vi "Read Host Stream.vi"(5 "Pause":bool, 7 "Init?":bool, 8 "error in (no error)":errorcluster, 10 "Sort By ID":bool, 11 "Refs in":T2) -> (0 "error out":errorcluster, 2 "Stream":T1, 3 "Refs out":T2)   [LabVIEW 2019, in "CAN Streaming Support Workspace Shared.lvlib"]
uses:
  CAN Streaming Support Workspace Shared.lvlib
  Types/Host Stream API Refs.ctl
  <vilib>/xnet/xnet.llb/XNET CAN Comm.ctl
  <vilib>/xnet/xnet.llb/XNET CAN Comm State.ctl
  <vilib>/xnet/xnet.llb/XNET CAN Last Err.ctl
  <vilib>/xnet/xnet.llb/XNET Frame CAN.ctl
  <vilib>/xnet/xnet.llb/XNET Frame Type CAN.ctl
  Types/Host Stream API Data.ctl
  <userlib>/_OpenG.lib/array/array.llb/Sort Array__ogtk.vi
  <userlib>/_OpenG.lib/array/array.llb/Sort 2D Array (String)__ogtk.vi
  <resource>/objmgr/ni.dex.rc
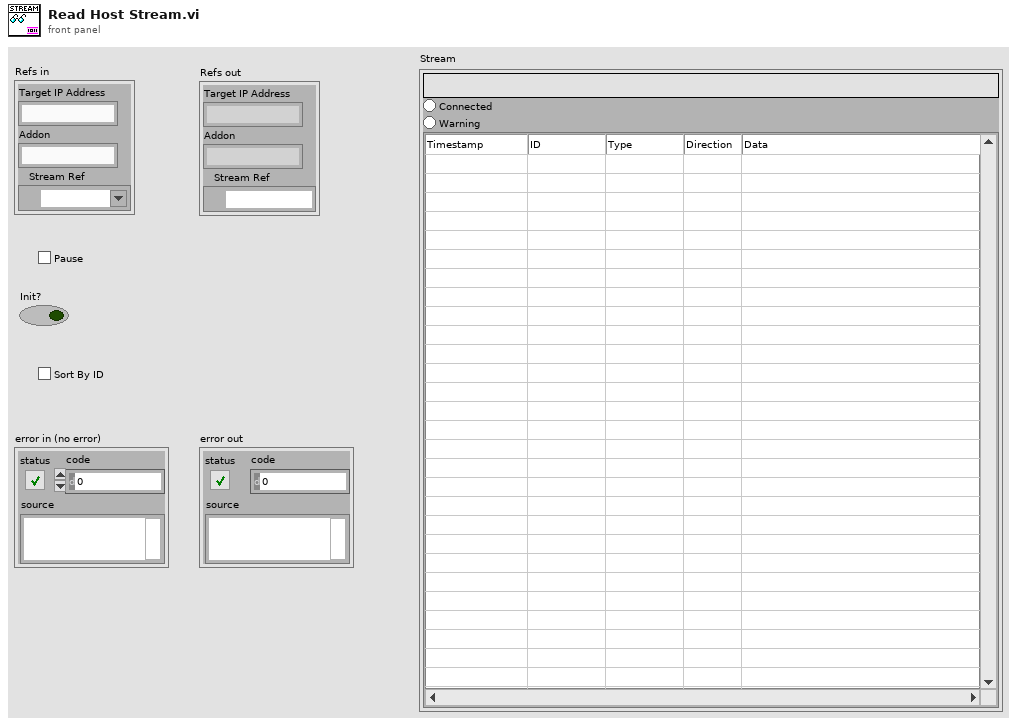
[diagram p1: front panel]
types:
  T1 = typedef "CAN Streaming Support Workspace Shared.lvlib/Host Stream API Data.ctl" = cluster{"State":string, "Connected":bool, "Warning":bool, "Table":string[][]}
  T2 = typedef "CAN Streaming Support Workspace Shared.lvlib/Host Stream API Refs.ctl" = cluster{"Target IP Address":string, "Addon":string, "Stream Ref":refnum<k21>}
  T3 = typedef "XNET CAN Comm.ctl" = cluster{"fault code":i32, "fault?":bool, "communication state":T4, "last error":T5, "receive error counter":u8, "transmit error counter":u8, "transceiver error?":bool, "sleep?":bool}
  T4 = typedef "XNET CAN Comm State.ctl" = u8
  T5 = typedef "XNET CAN Last Err.ctl" = u8
  T6 = typedef "XNET Frame CAN.ctl" = cluster{"timestamp":timestamp, "payload":u8[], "identifier":u32, "type":T7, "extended?":bool, "echo?":bool}
  T7 = typedef "XNET Frame Type CAN.ctl" = u8
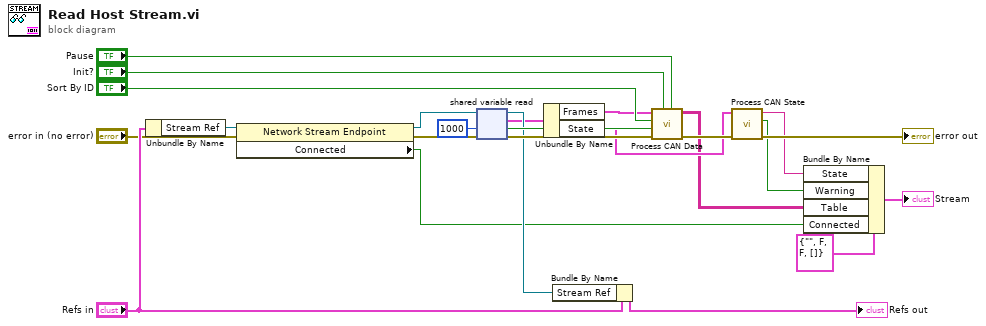
[diagram p0: block diagram]
diagram:
  n1 = Unbundle By Name("Refs in") -> ("Stream Ref"=w16:refnum<k21>)
  n2 = property class="Network Stream Endpoint"(reference=w16, error in="error in (no error)") -> (reference out=w13:refnum<k21>, error out=w15:errorcluster, "Connected"=w2:bool)
  n3 = shared-variable-read(w13, w15, 1000 ("timeout ms")) -> (w18:refnum<k21>, w23:errorcluster, w22:bool, w8:cluster{"State":T3, "Frames":T6[]})
  n4 = Unbundle By Name(w8) -> ("Frames"=w11:T6[], "State"=w7:T3)
  n5 = Bundle By Name(cluster="Refs in", "Stream Ref"=w18) -> (→"Refs out":T2)
  n6 = call "Process CAN Data.vi"("Pause"="Pause", "Init?"="Init?", "error in (no error)"=w23, "Timed Out?"=w22, "Sort By ID"="Sort By ID", "CAN Frames (from XNET Read)"=w11) -> ("error out"=w10:errorcluster, "Output Array"=w1:string[][])  [unwired: 4 in]
  n7 = call "Process CAN State.vi"("error in (no error)"=w10, "State"=w7) -> ("error out"=→"error out":errorcluster, "Warning"=w3:bool, "State"=w4:string)  [unwired: 7 in]
  n8 = Bundle By Name(cluster=T1 {"State"="", "Connected"=FALSE, "Warning"=FALSE, "Table"=[]} ("Stream"), "State"=w4, "Warning"=w3, "Table"=w1, "Connected"=w2) -> (→"Stream":T1)
